vi "Read lockin configuration.vi"(0 "tdms file":refnum<k34>, 1 "Pipeline delay":dbl=28.0, 5 "group name in":string, 9 "Channel name":string, 11 "Error In":errorcluster, 12 "Sample rate":dbl=125000000.0 format="%#_6p", 13 "DDS phase modulus":u64=100000000 format="%x") -> (2 "dt":dbl, 3 "Frequency word":u32, 4 "tdms file out":refnum<k34>, 6 "Frequency":dbl format="%_19p", 8 "t0":timestamp, 10 "Phase":dbl, 14 "Phase word":u32, 15 "Error Out":errorcluster)   [LabVIEW 2015]
panel:
  out "Data out":waveform(dbl)
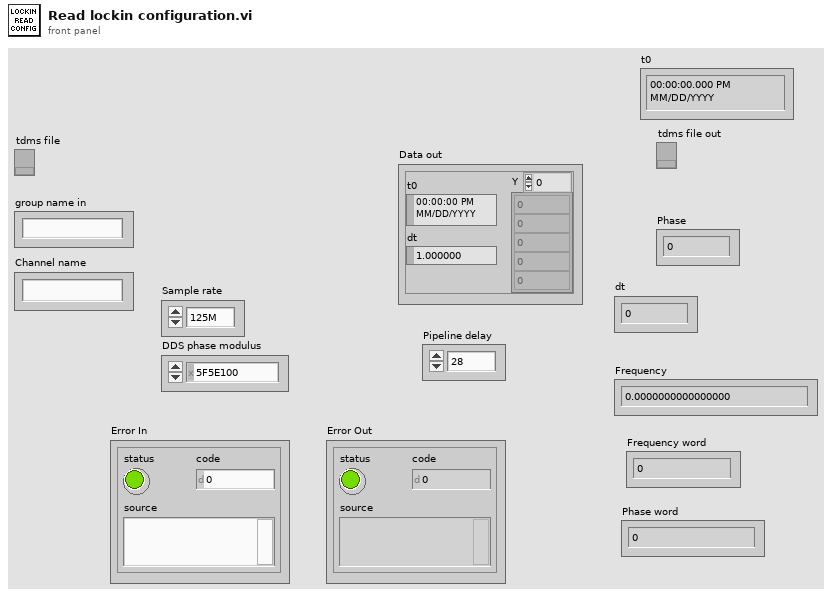
[diagram p1: front panel]
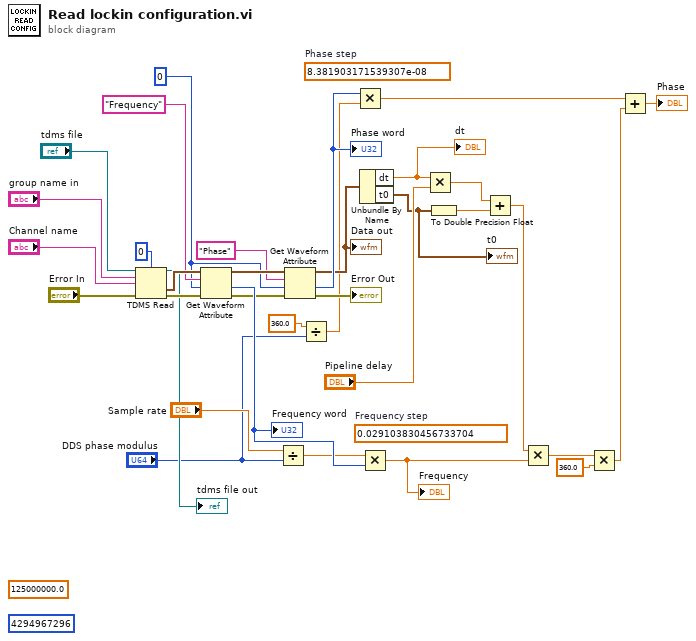
[diagram p0: block diagram]
diagram:
  w19 = u32 0 ("index")
  (unwired) 8.381903171539307e-08  # Phase step
  (unwired) 0.029103830456733704  # Frequency step
  (unwired) u64 4294967296
  (unwired) 125000000.0
  n1 = TDMS Read(0:"tdms file", 2:i64 0 ("count (-1: all)"), 5:"group name in", 7:"Channel name", 11:"Error In") -> (4:→"tdms file out":refnum<k34>, 10:w25:waveform(dbl), 15:w23:errorcluster)  [unwired: 3 in, 3 out]
  n2 = Get Waveform Attribute(4:w23, 5:w19, 6:"Frequency" ("name"), 7:w25) -> (0:w21:errorcluster, 1:w34:u32, 3:w22:waveform(dbl))  [unwired: 1 out]
  "Frequency word" <- w34
  n3 = Divide(x="Sample rate", y="DDS phase modulus") -> (x/y=w6:dbl)
  n4 = Get Waveform Attribute(4:w21, 5:w19, 6:"Phase" ("name"), 7:w22) -> (0:→"Error Out":errorcluster, 1:w33:u32, 3:w17:waveform(dbl))  [unwired: 1 out]
  "Phase word" <- w33
  "Data out" <- w17
  n5 = Divide(x=360.0, y="DDS phase modulus") -> (x/y=w3:dbl)
  n6 = Multiply(x=w33, y=w3) -> (x*y=w14:dbl)
  n7 = Unbundle By Name(w17) -> ("dt"=w1:dbl, "t0"=w2:timestamp)
  "t0" <- w2
  "dt" <- w1
  n8 = Multiply(x=w6, y=w34) -> (x*y=w32:dbl)
  "Frequency" <- w32
  n9 = Multiply(x=w1, y="Pipeline delay") -> (x*y=w26:dbl)
  n10 = To Double Precision Float(number=w2) -> (double precision float=w31:dbl)
  n11 = Add(x=w26, y=w31) -> (x+y=w27:dbl)
  n12 = Multiply(x=w27, y=w32) -> (x*y=w30:dbl)
  n13 = Multiply(x=w30, y=360.0) -> (x*y=w15:dbl)
  n14 = Add(x=w14, y=w15) -> (x+y=→"Phase":dbl)
